vi "Set Server Stop UE.vi"(10 "Server Stop":refnum<user-event>, 11 "OOP Server in":refnum<class "Template Server.lvclass">) -> (3 "OOP Server out":refnum<class "Template Server.lvclass">)   [LabVIEW 2019, in "Template Server.lvlib" / "Template Server.lvclass"]
uses:
  Template Server.lvclass
  Template Server.lvclass/Template Server.ctl
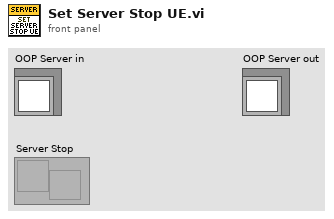
[diagram p1: front panel]
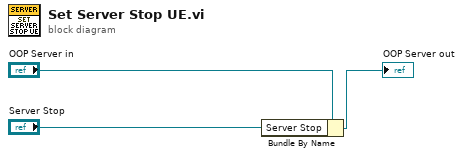
[diagram p0: block diagram]
diagram:
  n1 = Bundle By Name(cluster="OOP Server in", "Server Stop"="Server Stop") -> (→"OOP Server out":refnum<class "Template Server.lvclass">)
